vi "New VI Icon Canvas.vi"(8 "error in (no error)":errorcluster, 11 "VI Ref (Caller)":refnum<vi>) -> (0 "error out":errorcluster, 3 "VI Icon Canvas out":refnum<class "VI Icon Canvas.lvclass">)   [LabVIEW 2020, in "Glyph Drawer.lvlib" / "VI Icon Canvas.lvclass"]
uses:
  VI Icon Canvas.lvclass
  VI Icon Canvas.lvclass/VI Icon Canvas.ctl
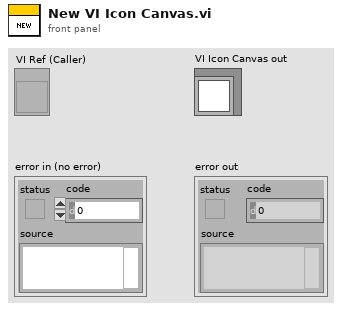
[diagram p1: front panel]
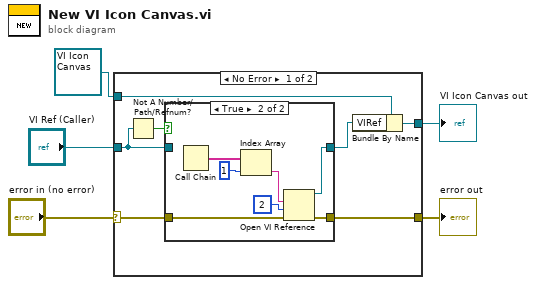
[diagram p0: block diagram]
diagram:
  n1 = case shown="No Error" "error in (no error)" {
    selector: "error in (no error)" -> [w7 w23]
    tunnel: [w6 w23] -> w4
    tunnel: [w11 w22] -> w2
    tunnel: refnum<class "VI Icon Canvas.lvclass"> refnum ("VI Icon Canvas in") -> [w12 w22]
    tunnel: "VI Ref (Caller)" -> [w8 _]
    frame No Error {
      n2 = Not A Number/Path/Refnum?(number/path/refnum=w8) -> (NaN/Path/Refnum?=w10:bool)
      n3 = case shown="True" w10 {
        tunnel: [w14 w17] -> w9
        tunnel: w8 -> [w14 _]
        tunnel: w7 -> [w13 w16]
        tunnel: [w13 w15] -> w6
        frame False {
        }
        frame True {
          n4 = Call Chain() -> (call chain=w18:string[])
          n5 = Index Array(array=w18, index=1 ("Index")) -> (element=w20:string)
          n6 = Open VI Reference(vi path=w20, options=2, error in (no error)=w16) -> (vi reference=w17:refnum<vi>, error out=w15:errorcluster)  [unwired: 3 in]
        }
      }
      n7 = Bundle By Name(cluster=w12, "VIRef"=w9) -> (w11:refnum<class "VI Icon Canvas.lvclass">)
    }
    frame Error {
    }
  }
  "error out" <- w4
  "VI Icon Canvas out" <- w2
